vi "Enqueue.vi"(8 "error in (no error)":errorcluster, 9 "Message Priority (Normal)":T1=enum."Normal", 10 "Message":refnum<class "Message.lvclass">, 11 "Message Enqueuer in":refnum<class "Message Enqueuer.lvclass">) -> (0 "error out":errorcluster, 3 "Message Enqueuer out":refnum<class "Message Enqueuer.lvclass">)   [LabVIEW 2020, in "Actor Framework.lvlib" / "Message Enqueuer.lvclass"]
doc: "(<B>Filename</B>: Actor Framework.lvlib:Message Enqueuer.lvclass:Enqueue.vi)\n\nSends a message."
uses:
  <vilib>/ActorFramework/Message Enqueuer/Message Enqueuer.lvclass
  <vilib>/ActorFramework/Message/Message.lvclass
  <vilib>/ActorFramework/Message Enqueuer/Message Priority.ctl
  <vilib>/ActorFramework/Message Enqueuer/Message Enqueuer.lvclass/Message Enqueuer.ctl
  <vilib>/ActorFramework/Message Priority Queue/Message Priority Queue.lvclass
  <resource>/AFDebug/AF Debug.lvlib
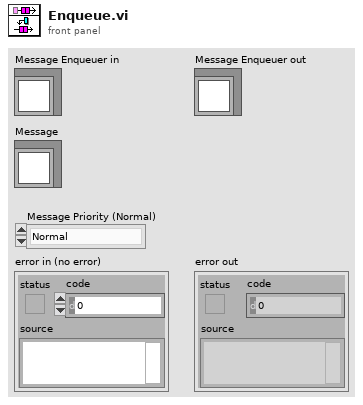
[diagram p1: front panel]
types:
  T1 = typedef "Actor Framework.lvlib/Message Enqueuer.lvclass/Message Priority.ctl" = enum16{"Low", "Normal", "High"}
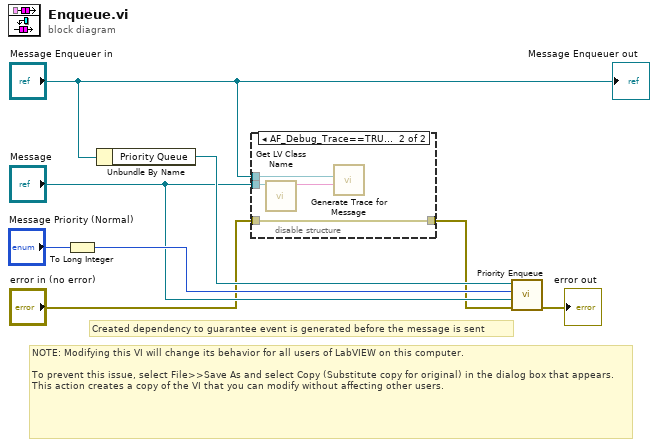
[diagram p0: block diagram]
diagram:
  # "Created dependency to guarantee event is generated before the message is sent"
  # "NOTE: Modifying this VI will change its behavior for all users of LabVIEW on this computer.\n\nTo prevent this issue, select File>>Save As and select Copy (Substitute copy for original) in the dialog box that appears. This action creates a copy of the VI that you can modify without affecting other users."
  n1 = To Long Integer(number="Message Priority (Normal)") -> (32bit integer=w6:i32)
  n2 = Unbundle By Name("Message Enqueuer in") -> ("Priority Queue"=w8:refnum<class "Message Priority Queue.lvclass">)
  n3 = disable-structure shown="AF_Debug_Trace==TRUE" {
    disable-tunnel: "error in (no error)" -> [w9 w13]
    disable-tunnel: [w9 w13] -> w1
    disable-tunnel: "Message Enqueuer in" -> [_ w11]
    disable-tunnel: "Message" -> [_ w10]
    frame condition #0 (active) {
    }
    frame condition #1 {
      n4 = call <vilib>:"Get LV Class Name.vi"("object"=w10) -> ("class name"=w12:string)  [unwired: 9 in, 1 out]
      n5 = call <resource>:"Generate Trace for Message.vi"("Message Name"=w12, "Receiver Enqueuer"=w11) -> ()  [unwired: 10 in]
    }
  }
  n6 = call <vilib>:"Priority Enqueue.vi"("error in (no error)"=w1, "Message"="Message", "priority"=w6, "Priority Queue in"=w8) -> ("error out"=→"error out":errorcluster)  [unwired: 6 in, 1 out]
  "Message Enqueuer out" <- "Message Enqueuer in"
